vi "05TRM800_MPHINC.vi"(4 "MPH DOWN":bool, 5 "MPH UP":bool, 6 "INC DOWN":bool, 7 "INC UP":bool, 8 "error in (no error)":errorcluster, 11 "Enum":enum16{"Initialize", "Set"}(ring)) -> (0 "error out":errorcluster, 2 "INC":dbl, 3 "MPH":dbl)   [LabVIEW 2015]
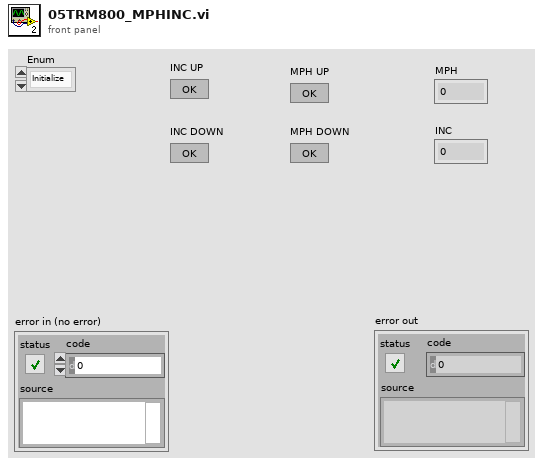
[diagram p1: front panel]
types:
  T1 = enum16{"Initialize", "Next", "Send RSET", "Set MPH", "Set INC", "Part to 0"}
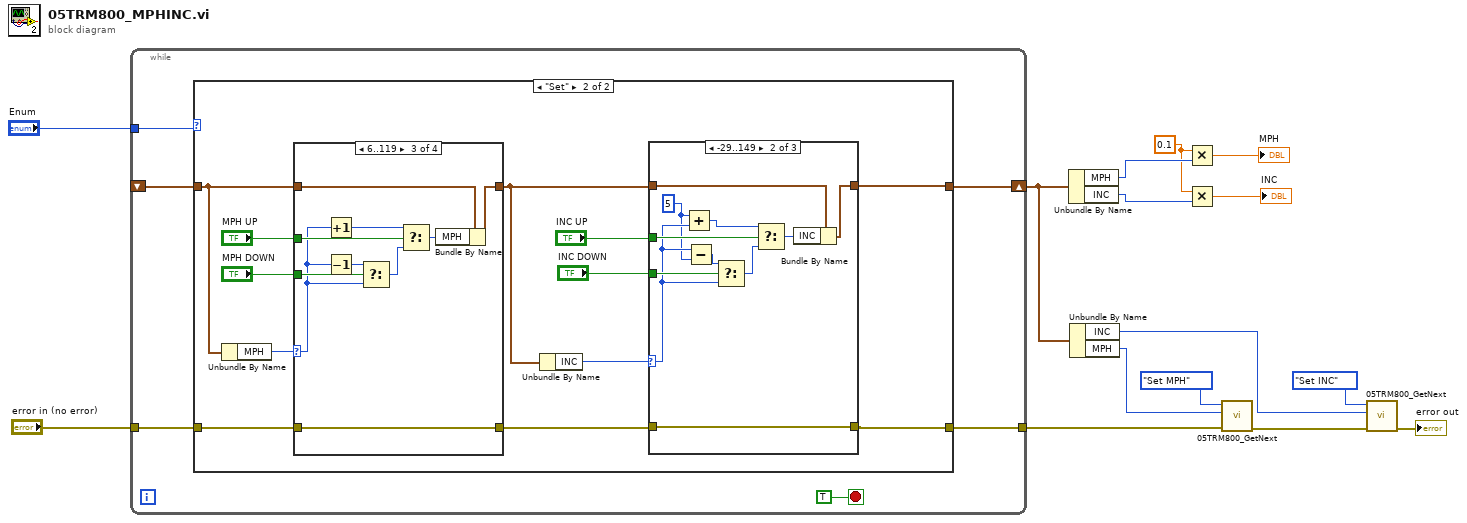
[diagram p0: block diagram]
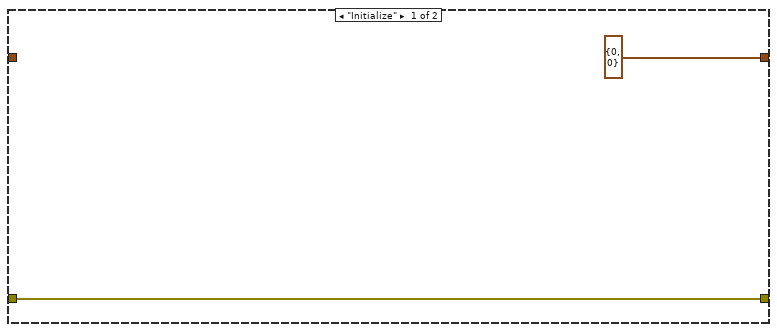
[diagram p2: hidden frame]
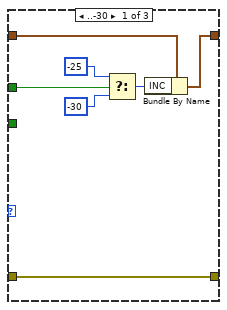
[diagram p3: hidden frame]
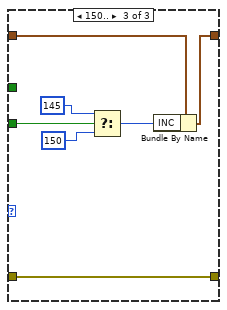
[diagram p4: hidden frame]
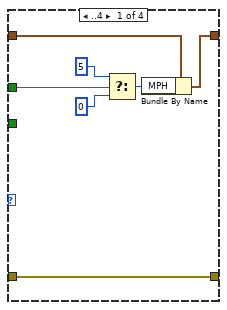
[diagram p5: hidden frame]
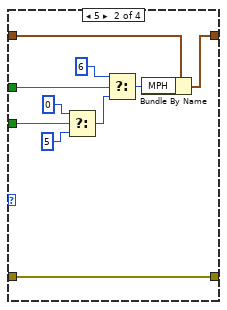
[diagram p6: hidden frame]
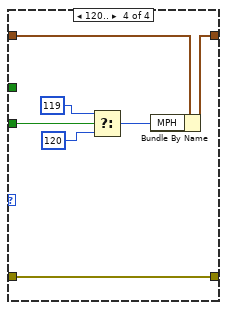
[diagram p7: hidden frame]
diagram:
  w11 = 0.1 ("x")
  n1 = while {
    tunnel: "error in (no error)" -> [w20]
    tunnel: [w19] -> w5
    tunnel: "Enum" -> [w18]
    shift-right: [w17] -> w8
    shift-left: _ -> [w16]
    stop <- TRUE stop-if-true
    n2 = case shown="\"Set\"" w18 {
      tunnel: w20 -> [w23 w35]
      tunnel: [w23 w26] -> w19
      tunnel: [cluster{"MPH":i32, "INC":i32} {"MPH"=0, "INC"=0} w25] -> w17
      tunnel: w16 -> [_ w33]
      frame "Initialize" {
      }
      frame "Set" {
        n3 = Unbundle By Name(w33) -> ("MPH"=w34:i32)
        n4 = case shown="6..119" w34 {
          selector: w34 -> [_ _ w79 _]
          tunnel: w35 -> [w67 w77 w87 w94]
          tunnel: [w67 w77 w87 w94] -> w30
          tunnel: w33 -> [w65 w75 w85 w92]
          tunnel: "MPH UP" -> [w64 w74 w84 _]
          tunnel: "MPH DOWN" -> [_ w70 w81 w91]
          tunnel: [w66 w76 w86 w93] -> w29
          frame ..4 {
            n5 = Select(t=5 ("MPH"), s=w64, f=0 ("MPH")) -> (s? t:f=w63:i32)
            n6 = Bundle By Name(cluster=w65, "MPH"=w63) -> (w66:cluster{"MPH":i32, "INC":i32})
          }
          frame 5 {
            n7 = Select(t=0 ("MPH"), s=w70, f=5 ("MPH")) -> (s? t:f=w71:i32)
            n8 = Select(t=6 ("MPH"), s=w74, f=w71) -> (s? t:f=w73:i32)
            n9 = Bundle By Name(cluster=w75, "MPH"=w73) -> (w76:cluster{"MPH":i32, "INC":i32})
          }
          frame 6..119 {
            n10 = Increment(x=w79) -> (x+1=w78:i32)
            n11 = Decrement(x=w79) -> (x-1=w80:i32)
            n12 = Select(t=w80, s=w81, f=w79) -> (s? t:f=w82:i32)
            n13 = Select(t=w78, s=w84, f=w82) -> (s? t:f=w83:i32)
            n14 = Bundle By Name(cluster=w85, "MPH"=w83) -> (w86:cluster{"MPH":i32, "INC":i32})
          }
          frame 120.. {
            n15 = Select(t=119 ("MPH"), s=w91, f=120) -> (s? t:f=w90:i32)
            n16 = Bundle By Name(cluster=w92, "MPH"=w90) -> (w93:cluster{"MPH":i32, "INC":i32})
          }
        }
        n17 = Unbundle By Name(w29) -> ("INC"=w24:i32)
        n18 = case shown="-29..149" w24 {
          selector: w24 -> [_ w45 _]
          tunnel: w30 -> [w42 w53 w60]
          tunnel: [w42 w53 w60] -> w26
          tunnel: w29 -> [w40 w51 w58]
          tunnel: "INC UP" -> [w39 w50 _]
          tunnel: "INC DOWN" -> [_ w47 w57]
          tunnel: [w41 w52 w59] -> w25
          frame ..-30 {
            n19 = Select(t=-25 ("MPH"), s=w39, f=-30 ("MPH")) -> (s? t:f=w38:i32)
            n20 = Bundle By Name(cluster=w40, "INC"=w38) -> (w41:cluster{"MPH":i32, "INC":i32})
          }
          frame -29..149 {
            w44 = 5
            n21 = Add(x=w44, y=w45) -> (x+y=w46:i32)
            n22 = Subtract(x=w45, y=w44) -> (x-y=w43:i32)
            n23 = Select(t=w43, s=w47, f=w45) -> (s? t:f=w48:i32)
            n24 = Select(t=w46, s=w50, f=w48) -> (s? t:f=w49:i32)
            n25 = Bundle By Name(cluster=w51, "INC"=w49) -> (w52:cluster{"MPH":i32, "INC":i32})
          }
          frame 150.. {
            n26 = Select(t=145 ("MPH"), s=w57, f=150) -> (s? t:f=w56:i32)
            n27 = Bundle By Name(cluster=w58, "INC"=w56) -> (w59:cluster{"MPH":i32, "INC":i32})
          }
        }
      }
    }
  }
  n28 = Unbundle By Name(w8) -> ("MPH"=w13:i32, "INC"=w10:i32)
  n29 = Unbundle By Name(w8) -> ("INC"=w1:i32, "MPH"=w6:i32)
  n30 = Multiply(x=w11, y=w13) -> (x*y=→"MPH":dbl)
  n31 = Multiply(x=w11, y=w10) -> (x*y=→"INC":dbl)
  n32 = call "05TRM800_GetNext.vi"("error in (no error)"=w5, "Value"=w6, "Enum"=T1."Set MPH") -> ("error out"=w2:errorcluster)  [unwired: 7 in, 1 out]
  n33 = call "05TRM800_GetNext.vi"("error in (no error)"=w2, "Value"=w1, "Enum"=T1."Set INC") -> ("error out"=→"error out":errorcluster)  [unwired: 7 in, 1 out]
